vi "Write then flush.vi"(8 "error in (no error)":errorcluster, 10 "TX Data":string, 11 "Serial Device in":refnum<class "Serial Device.lvclass">) -> (0 "error out":errorcluster, 3 "Serial Device out":refnum<class "Serial Device.lvclass">)   [LabVIEW 2015, in "Serial Device.lvclass"]
uses:
  Serial Device.lvclass
  Serial Device.lvclass/Serial Device.ctl
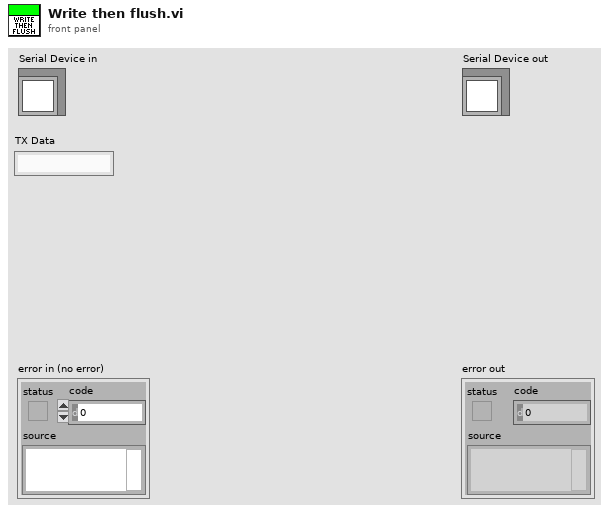
[diagram p1: front panel]
types:
  T1 = typedef "Semaphore RefNum" = refnum<k1>
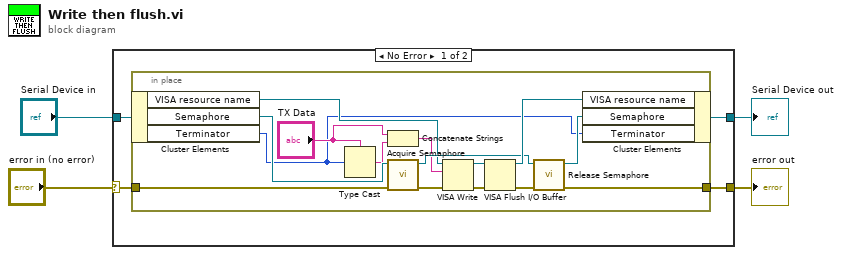
[diagram p0: block diagram]
diagram:
  n1 = case shown="No Error" "error in (no error)" {
    selector: "error in (no error)" -> [w8 w25]
    tunnel: [w5 w25] -> w3
    tunnel: [w6 w24] -> w1
    tunnel: "Serial Device in" -> [w7 w24]
    frame No Error {
      n2 = in-place {
        in-place-border: w8 -> [w23]
        in-place-border: [w17] -> w5
        n3 = in-place-cluster #1(w7) -> ("VISA resource name"=w15:refnum<visa-resource-name>, "Semaphore"=w22:T1, "Terminator"=w11:u8)
        n4 = Type Cast(type="TX Data", x=w11) -> (*(type *) &x=w12:string)
        n5 = Concatenate Strings("TX Data", w12) -> (w14:string)
        n6 = call <vilib>:"Acquire Semaphore.vi"("error in (no error)"=w23, "semaphore"=w22) -> ("error out"=w16:errorcluster, "semaphore out"=w18:T1)  [unwired: 3 in, 1 out]
        n7 = VISA Write(VISA resource name=w15, write buffer=w14, error in (no error)=w16) -> (VISA resource name out=w10:refnum<visa-resource-name>, error out=w9:errorcluster)  [unwired: 1 out]
        n8 = VISA Flush I/O Buffer(VISA resource name=w10, error in (no error)=w9) -> (VISA resource name out=w21:refnum<visa-resource-name>, error out=w20:errorcluster)  [unwired: 1 in]
        n9 = call <vilib>:"Release Semaphore.vi"("error in (no error)"=w20, "semaphore"=w18) -> ("error out"=w17:errorcluster, "semaphore out"=w19:T1)  [unwired: 4 in]
        n10 = in-place-cluster #1("VISA resource name"=w21, "Semaphore"=w19, "Terminator"=w11) -> (w6:refnum<class "Serial Device.lvclass">)
      }
    }
    frame Error {
    }
  }
  "error out" <- w3
  "Serial Device out" <- w1
